vi "Accumulate(DBL).vi"(7 "enable":bool=TRUE, 8 "error in":errorcluster, 9 "reset":bool, 11 "input":dbl) -> (0 "error out":errorcluster, 3 "accumulation":dbl)   [LabVIEW 2012, in "Accumulate.lvlib"]
uses:
  Accumulate.lvlib
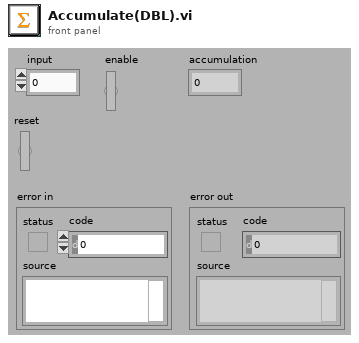
[diagram p1: front panel]
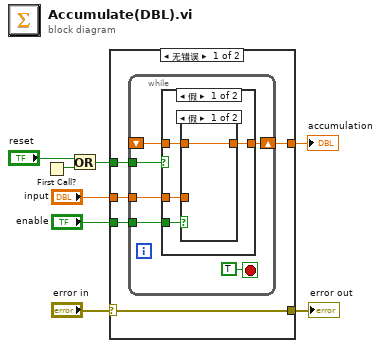
[diagram p0: block diagram]
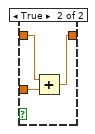
[diagram p2: hidden frame]
diagram:
  n1 = First Call?() -> (First Call?: T/F=w3:bool)
  n2 = Or(x="reset", y=w3) -> (x .or. y?=w1:bool)
  n3 = case shown="无错误" "error in" {
    selector: "error in" -> [w13 w29]
    tunnel: [w13 w29] -> w8
    tunnel: [w12 _] -> w6
    tunnel: "enable" -> [w11 _]
    tunnel: "input" -> [w10 _]
    tunnel: w1 -> [w9 _]
    frame No Error {
      n4 = while {
        shift-right: [w17] -> w12
        shift-left: _ -> [w18]
        tunnel: w11 -> [w16]
        tunnel: w10 -> [w15]
        tunnel: w9 -> [w14]
        stop <- TRUE stop-if-true
        n5 = case shown="假" w14 {
          tunnel: [w20 w28] -> w17
          tunnel: w16 -> [w23 _]
          tunnel: w15 -> [w22 w28]
          tunnel: w18 -> [w21 _]
          frame False {
            n6 = case shown="假" w23 {
              tunnel: w22 -> [_ w27]
              tunnel: w21 -> [w24 w26]
              tunnel: [w24 w25] -> w20
              frame False {
              }
              frame True {
                n7 = Add(x=w26, y=w27) -> (x+y=w25:dbl)
              }
            }
          }
          frame True {
          }
        }
      }
    }
    frame Error {
    }
  }
  "error out" <- w8
  "accumulation" <- w6
